vi "causal Delay.vi"(0 "DELAY":i32(knob) scale=-10.0..100.0, 2 "X":dbl[](array[numeric]) format="%0.2f") -> (1 "Delayed sequence":dbl[](array[numeric]) format="%0.2f")   [LabVIEW 2009]
uses:
  <vilib>/Analysis/2dsp.llb/1D Convolution (DBL).vi
  <vilib>/Analysis/NI_AALBase.lvlib
  <vilib>/Analysis/NI_AALPro.lvlib
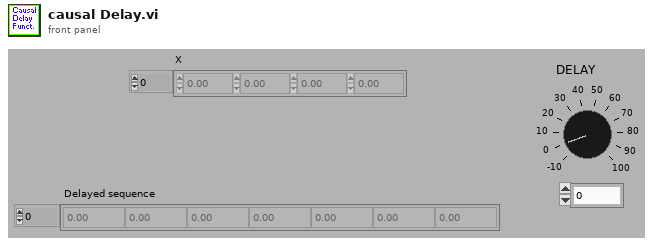
[diagram p1: front panel]
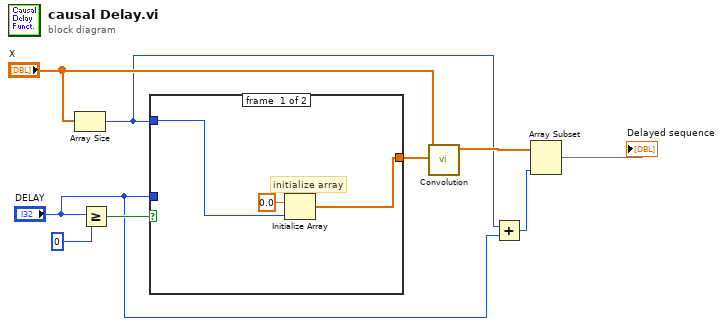
[diagram p0: block diagram]
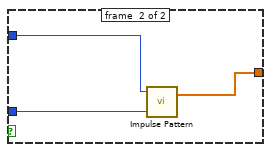
[diagram p2: hidden frame]
diagram:
  n1 = Array Size(array="X") -> (size(s)=w3:i32)
  n2 = Greater Or Equal?(x="DELAY", y=0) -> (x >= y?=w8:bool)
  n3 = case shown="True" w8 {
    tunnel: "DELAY" -> [_ w15]
    tunnel: [w11 w14] -> w6
    tunnel: w3 -> [w10 w13]
    frame #0 {
      # "initialize array"
      n4 = Initialize Array(0.0 ("element"), w10) -> (w11:dbl[])
    }
    frame #1 {
      n5 = call <vilib>:"Impulse Pattern.vi"("delay"=w15, "samples"=w13) -> ("Impulse Pattern"=w14:dbl[])  [unwired: 1 in, 1 out]
    }
  }
  n6 = call-poly <vilib>:"Convolution.vi"("Y"=w6, "X"="X") -> ("X * Y"=w5:dbl[])  [unwired: 8 in, 1 out]
  n7 = Add(x=w3, y="DELAY") -> (x+y=w2:i32)
  n8 = Array Subset(array=w5, length=w2) -> (→"Delayed sequence":dbl[])  [unwired: 1 in]
